vi "Extract from StartEnd and Duration.vi"(8 "Error":errorcluster, 9 "Duration(S)":dbl, 10 "From End(f)\nFrom Beginning(t)":bool, 11 "WavBuf":refnum<class "WavBuf.lvclass">) -> (0 "Error Out":errorcluster, 2 "Waveform Out":T1, 3 "WavBuf Out":refnum<class "WavBuf.lvclass">)   [LabVIEW 2024, in "WavBuf.lvclass"]
uses:
  WavBuf.lvclass
  Universal Controls/Waveform_Data.ctl
  WavBuf.lvclass/WavBuf.ctl
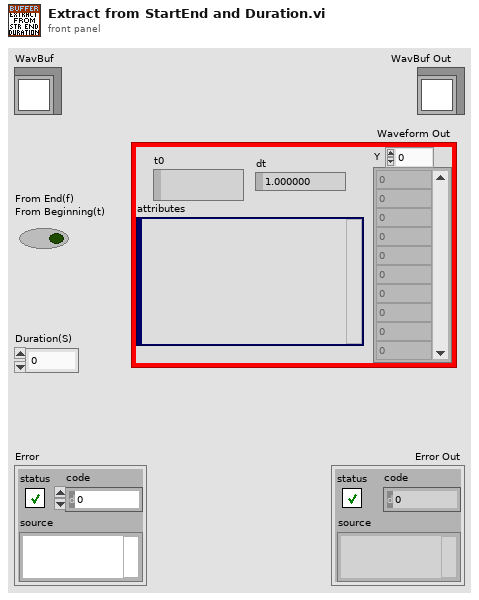
[diagram p1: front panel]
types:
  T1 = typedef "Waveform_Data.ctl" = waveform(dbl)
  T2 = typedef "Ref_DVR_Buffer.ctl" = refnum<data-value>
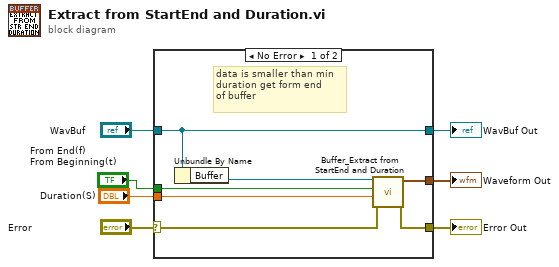
[diagram p0: block diagram]
diagram:
  n1 = case shown="No Error" "Error" {
    selector: "Error" -> [w9 w16]
    tunnel: [w13 w16] -> w6
    tunnel: [w11 w15] -> w4
    tunnel: "WavBuf" -> [w11 w15]
    tunnel: [w14 _] -> w3
    tunnel: "Duration(S)" -> [w12 _]
    tunnel: "From End(f)\nFrom Beginning(t)" -> [w8 _]
    frame No Error {
      # "data is smaller than min \nduration get form end \nof buffer"
      n2 = Unbundle By Name(w11) -> ("Buffer"=w10:T2)
      n3 = call "Buffer_Extract from StartEnd and Duration.vi"("Error"=w9, "Duration(S)"=w12, "From End(f)\nFrom Beginning(t)"=w8, "Buffer"=w10) -> ("Error Out"=w13:errorcluster, "Waveform Out"=w14:T1)  [unwired: 1 in, 5 out]
    }
    frame Error {
    }
  }
  "Error Out" <- w6
  "WavBuf Out" <- w4
  "Waveform Out" <- w3
